vi "coord2elipse.vi"(10 "diameter":dbl=10.0 format="%#_13g", 11 "Point Coordinates":cluster{"X":dbl, "Y":dbl}) -> (3 "Cluster":cluster{dbl, dbl, dbl, dbl})   [LabVIEW 2021, in "Framework_lib.lvlib"]
uses:
  QMH/Framework_lib.lvlib
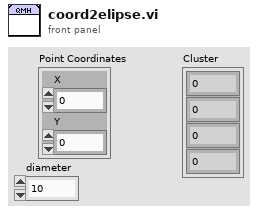
[diagram p1: front panel]
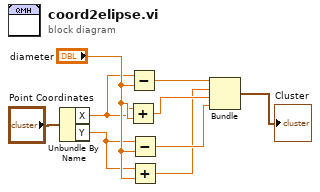
[diagram p0: block diagram]
diagram:
  n1 = Unbundle By Name("Point Coordinates") -> ("X"=w2:dbl, "Y"=w3:dbl)
  n2 = Add(x=w2, y="diameter") -> (x+y=w7:dbl)
  n3 = Subtract(x=w2, y="diameter") -> (x-y=w5:dbl)
  n4 = Subtract(x=w3, y="diameter") -> (x-y=w8:dbl)
  n5 = Add(x=w3, y="diameter") -> (x+y=w6:dbl)
  n6 = Bundle(w5, w6, w7, w8) -> (→"Cluster":cluster{dbl, dbl, dbl, dbl})  [unwired: 1 in]
